vi "Teleop.vi"(10 "Match Info":T4={"Autonomous Elapsed Seconds"=0.0, "TeleOp Elapsed Seconds"=0.0, "Disabled Elapsed Seconds"=0.0, "Visited Autonomous"=FALSE, "Visited TeleOp"=FALSE, "Visited Disabled"=FALSE, "Autonomous Settings"={"Autonomous Style"=enum."Independent", "VI Refnum"=refnum}}, 11 "Call Context":T5) -> ()   [LabVIEW 2016]
doc: "This VI is called for each TeleOp packet received from the DS where the robot is not disabled. It is often used to read from the joysticks and update I/O or to update setpoints for timed control loops. It should complete and return within 20 milliseconds or it may miss DS packets."
uses:
  <vilib>/Rock Robotics/WPI/DriverStation/WPI_DriverStationDerivedRobotMode.ctl
  <vilib>/Rock Robotics/WPI/DriverStation/WPI_DriverStationMatch Info.ctl
  <vilib>/Rock Robotics/WPI/ThirdParty/CanMotor/TalonSRX/CTRE_CANTalonSRX_VelocityMeasurementPeriod.ctl
  <vilib>/Rock Robotics/WPI/ThirdParty/CanMotor/TalonSRX/WPI_CANTalonSRX_BrakeOverride.ctl
  <vilib>/Rock Robotics/WPI/ThirdParty/CanMotor/TalonSRX/WPI_CANTalonSRX_APIControlMode.ctl
  <vilib>/Rock Robotics/WPI/Utilities/WPI_GetSetVariantRefNum.vi
  <vilib>/Rock Robotics/Network Tables/NT Write Numeric Array.vi
  <vilib>/Rock Robotics/Network Tables/NT Write Boolean Array.vi
  <vilib>/Rock Robotics/Network Tables/NT Write Number.vi
  <vilib>/Rock Robotics/Network Tables/NT Read Boolean.vi
  <vilib>/Rock Robotics/Network Tables/NT Read Number.vi
  Robot Global Data.vi
panel:
  in  "Gear speed":dbl=2.0
  in  "Servo Disengaged Pos":dbl
  in  "Servo Engaged Pos":dbl
  in  "Disable Flash":bool=TRUE
  out "Display Mode":T1(ring)
  out "Color":T2(ring)
  out "Servo Position":dbl
  out "Error Left":dbl
  out "Error Right":dbl
  in  "P Shooting":dbl=0.08
  in  "Shooter \n%VBus":dbl
  out "Left Drive RPM":cluster{"Sensor Velocity":dbl, dbl}(graph)
  out "Right Drive RPM":cluster{"Sensor Velocity":dbl, dbl}(graph)
  out "Left RPM":dbl
  out "Right RPM":dbl
  in  "Shoot":bool
  out "DISABLED":bool
  out "Right FPS":dbl
  out "Left FPS":dbl
  in  "Velocity Measurement Period":T3=1 items=["Period_1ms"=1, "Period_2ms"=2, "Period_5ms"=5, "Period_10ms"=10, "Period_20ms"=20, "Period_25ms"=25, "Period_50ms"=50, "Period_100ms"=100]
  in  "Velocity Sample Window":u32=100
  out "Background":bool
  out "Shooter RPM":dbl
  out "Velocity":cluster{"Sensor Velocity":dbl, "Output":dbl}(graph)
  in  "P":dbl=0.0125
  in  "I":dbl
  in  "D":dbl
  in  "F":dbl=0.167
  in  "I Zone":dbl
  in  "Ramp Rate":dbl
  # "Shooter Speed Settings"
  # "Shooter Options"
  # "LED Status"
  # "Servo"
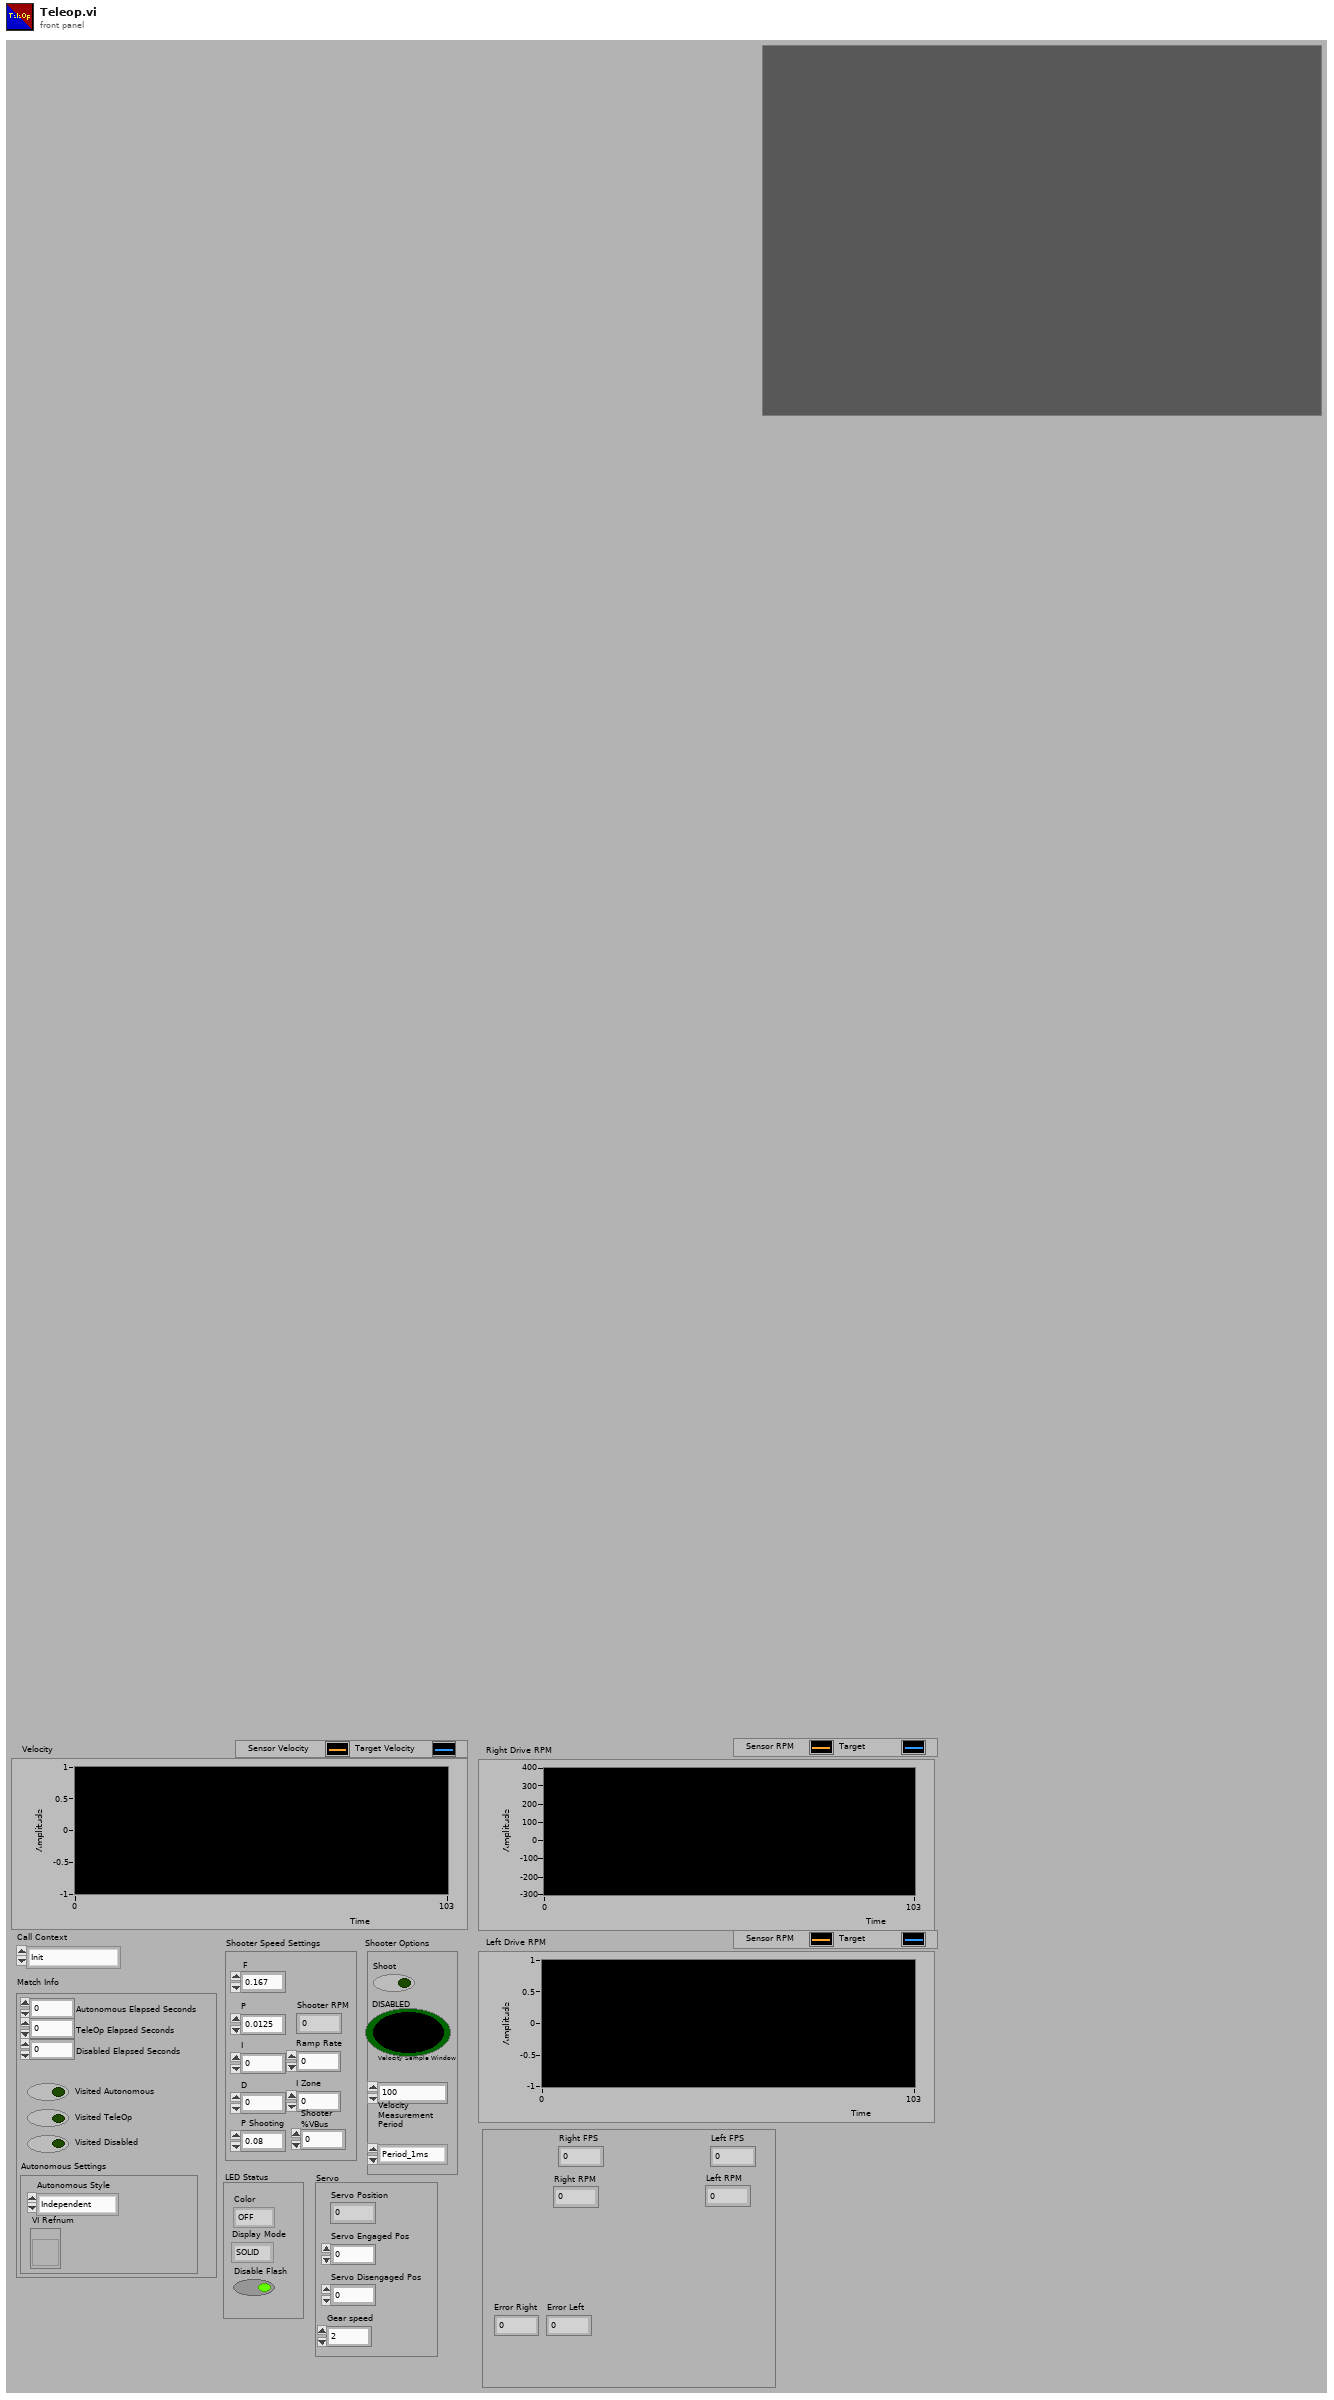
[diagram p1: front panel]
types:
  T1 = enum16{"SOLID", "FLASH 500ms", "FLASH 1000ms", "OFF"}
  T2 = enum16{"OFF", "RED", "GREEN", "BLUE", "PURPLE", "YELLOW", "TEAL", "WHITE", "RAINBOW"}
  T3 = typedef "CTRE_CANTalonSRX_VelocityMeasurementPeriod.ctl" = u16
  T4 = typedef "WPI_DriverStationMatch Info.ctl" = cluster{"Autonomous Elapsed Seconds":dbl, "TeleOp Elapsed Seconds":dbl, "Disabled Elapsed Seconds":dbl, "Visited Autonomous":bool, "Visited TeleOp":bool, "Visited Disabled":bool, "Autonomous Settings":cluster{"Autonomous Style":enum16{"Iterative", "Independent"}, "VI Refnum":refnum<vi>}}
  T5 = typedef "WPI_DriverStationDerivedRobotMode.ctl" = enum16{"Init", "Execute", "Stop"}
  T6 = typedef "WPI_CANTalonSRX_APIControlMode.ctl" = enum8{"Percent VBus", "Speed", "Position", "Slave", "Unchanged / Invalid", "Voltage Compensation", "Current", "Motion Profile", "Motion Magic"}
  T7 = typedef "WPI_CANTalonSRX_BrakeOverride.ctl" = enum8{"No Override", "Override to Coast", "Override to Brake"}
  T8 = cluster{"Shooter":cluster{"Shoot":bool, "%VBus":dbl, "Shoot Trigger":dbl, "Target Rpm":dbl}, "Drive":cluster{"Drive Stright":bool, "Left Throttle":dbl, "Right Throttle":dbl, "Curve Power":dbl}, "Intake":cluster{"Invert":bool, "%VBus":dbl}, "Gear/Climb":cluster{"Invert":bool, "%VBus":dbl}, "Teleop Front Pannel":cluster{"Overide?":bool}}
  T9 = typedef "WPI_JoystickDevRef.ctl" = cluster{"Device":T10}
  T10 = typedef "WPI_JoystickDeviceEnum.ctl" = enum16{"USB 0", "USB 1", "USB 2", "USB 3", "USB 4", "USB 5"}
  T11 = typedef "CTRE_PigeonIMU_DeviceRef.ctl" = cluster{"DeviceStatus":errorcluster, "Device Number":u8, "Type":T12, "Device ID":u32}
  T12 = typedef "CTRE_PigeonIMU_ConnectionType.ctl" = u32
  T13 = typedef "CTRE_PigeonIMU_GlobalStatus.ctl" = cluster{"PigeonState":T14, "FusedHeading":cluster{"Heading":dbl, "Valid?":bool, "Fusing?":bool}, "YPR":cluster{"Yaw":dbl, "Pitch":dbl, "Roll":dbl}, "Compass":cluster{"Heading":dbl, "Magnitude":dbl, "Absolute Heading":dbl}, "Accelerometer":cluster{"Biased":cluster{"X":i16, "Y":i16, "Z":i16, "Norm":i16}, "Angles":cluster{"XZ Tilt":dbl, "YZ Tilt":dbl, "XY Tilt":dbl}}, "Magnetometer":cluster{"Raw":cluster{"X":i16, "Y":i16, "Z":i16}, "Biased":cluster{"X":i16, "Y":i16, "Z":i16}}, "Gyro":cluster{"X":dbl, "Y":dbl, "Z":dbl, "Norm":dbl}, "6D Quaternian":cluster{"W":dbl, "X":dbl, "Y":dbl, "Z":dbl}, "Temp. (C)":dbl, "UpTime":u32, "StartupStatus":cluster{"ResetCount":i32, "ResetFlags":i32, "FirmwareVersion":i32, "HasReset?":bool}, "Calibration":cluster{"CurrentMode":T15, "LastCalError":i32, "CalBooting?":bool}, "CAN Error":errorcluster, "AccumGyro":cluster{"X":dbl, "Y":dbl, "Z":dbl}, "Usage Frame":u32}
  T14 = typedef "CTRE_PigeonIMU_PigeonState.ctl" = enum16{"NoComm", "Initializing", "Ready", "UserCalibration"}
  T15 = typedef "CTRE_PigeonIMU_CalibrationMode.ctl" = u16
  T16 = typedef "WPI_PotentiometerDevRef.ctl" = cluster{"DevStatus":errorcluster, "Analog Channel":T17, "Invert Output":bool}
  T17 = typedef "FPGA_AIChannel.ctl" = enum8{"AI 0", "AI 1", "AI 2", "AI 3", "AI MXP 0", "AI MXP 1", "AI MXP 2", "AI MXP 3", "Invalid"}
  T18 = typedef "WPI_MotorControlDeviceRef.ctl" = cluster{"DeviceStatus":errorcluster, "Type":T19, "PWM":cluster{"PWM Channel":T20, "DeadBand":T21}, "CAN":cluster{"Device Number":u8, "SetOutput VI Ref":variant, "GetOutput VI Ref":variant, "Enable VI Ref":variant, "Disable VI Ref":variant, "Data":variant}, "Invert":bool}
  T19 = typedef "WPI_MotorControlType.ctl" = enum16{"PWM", "CAN"}
  T20 = typedef "FPGA_DIOPWMChannel.ctl" = enum8{"PWM 0", "PWM 1", "PWM 2", "PWM 3", "PWM 4", "PWM 5", "PWM 6", "PWM 7", "PWM 8", "PWM 9", "PWM MXP 0", "PWM MXP 1", "PWM MXP 2", "PWM MXP 3", "PWM MXP 4", "PWM MXP 5", "PWM MXP 6", "PWM MXP 7", "PWM MXP 8", "PWM MXP 9", "Invalid"}
  T21 = typedef "WPI_PWMDeadband.ctl" = cluster{"Name":string, "maxPositivePwm":i32, "minPositivePwm":i32, "centerPwm":i32, "maxNegativePwm":i32, "minNegativePwm":i32, "angularRange":u16}
  T22 = typedef "WPI_ServoDeviceRef.ctl" = cluster{"DeviceStatus":errorcluster, "PWM Channel":T20, "DeadBand":T21}
  T23 = typedef "WPI_CANTalonSRX_GlobalStatus.ctl" = cluster{"Applied Throttle":dbl, "Module Enabled":bool, "CAN Error":errorcluster, "Closed Loop Error":dbl, "Forward Limit Switch Closed":bool, "Reverse Limit Switch Closed":bool, "Sensor Position":dbl, "Sensor Velocity":dbl, "Current":dbl, "Sticky Fault - Over Temp":bool, "Sticky Fault - Under Voltage":bool, "Sticky Fault - Forward Limit":bool, "Sticky Fault - Reverse Limit":bool, "Sticky Fault - Forward Soft Limit":bool, "Sticky Fault - Reverse Soft Limit":bool, "Brake is Enabled":bool, "Encoder Position":dbl, "Encoder Velocity":dbl, "Encoder Index Count":dbl, "Encoder A Pin State":bool, "Encoder B Pin State":bool, "Encoder Index Pin State":bool, "Analog In":dbl, "Analog In Velocity":dbl, "Temperature (C)":dbl, "Battery Voltage":dbl, "Control 5 Is Supported":bool, "Current Profile Slot Select":dbl, "Pos Div 8":bool, "Vel Div 4":bool, "Pulse Width Position":i32, "Pulse Width Velocity":i32, "Pulse Width Rise To Rise (us)":i32, "Pulse Width Rise To Fall (us)":i32, "Mot Prof Active Is Under Run":bool, "Mot Prof Active Has Under Run":bool, "Mot Prof Active Is Last":bool, "Mot Prof Active Velocity Only":bool, "Mot Prof Active Is Valid":bool, "Mot Prof Buffer Is Full":bool, "Mot Prof Active Profile Slot Select":i32, "Mot Prof NextID":i32, "Mot Prof Count":i32, "Mot Prof Active Velocity":dbl, "Mot Prof Active Position":dbl, "Mot Prof Output Enable":i32, "UsageFrame":u32, "Motion Magic Active Trajectory":cluster{"Velocity":dbl, "Position":dbl}}
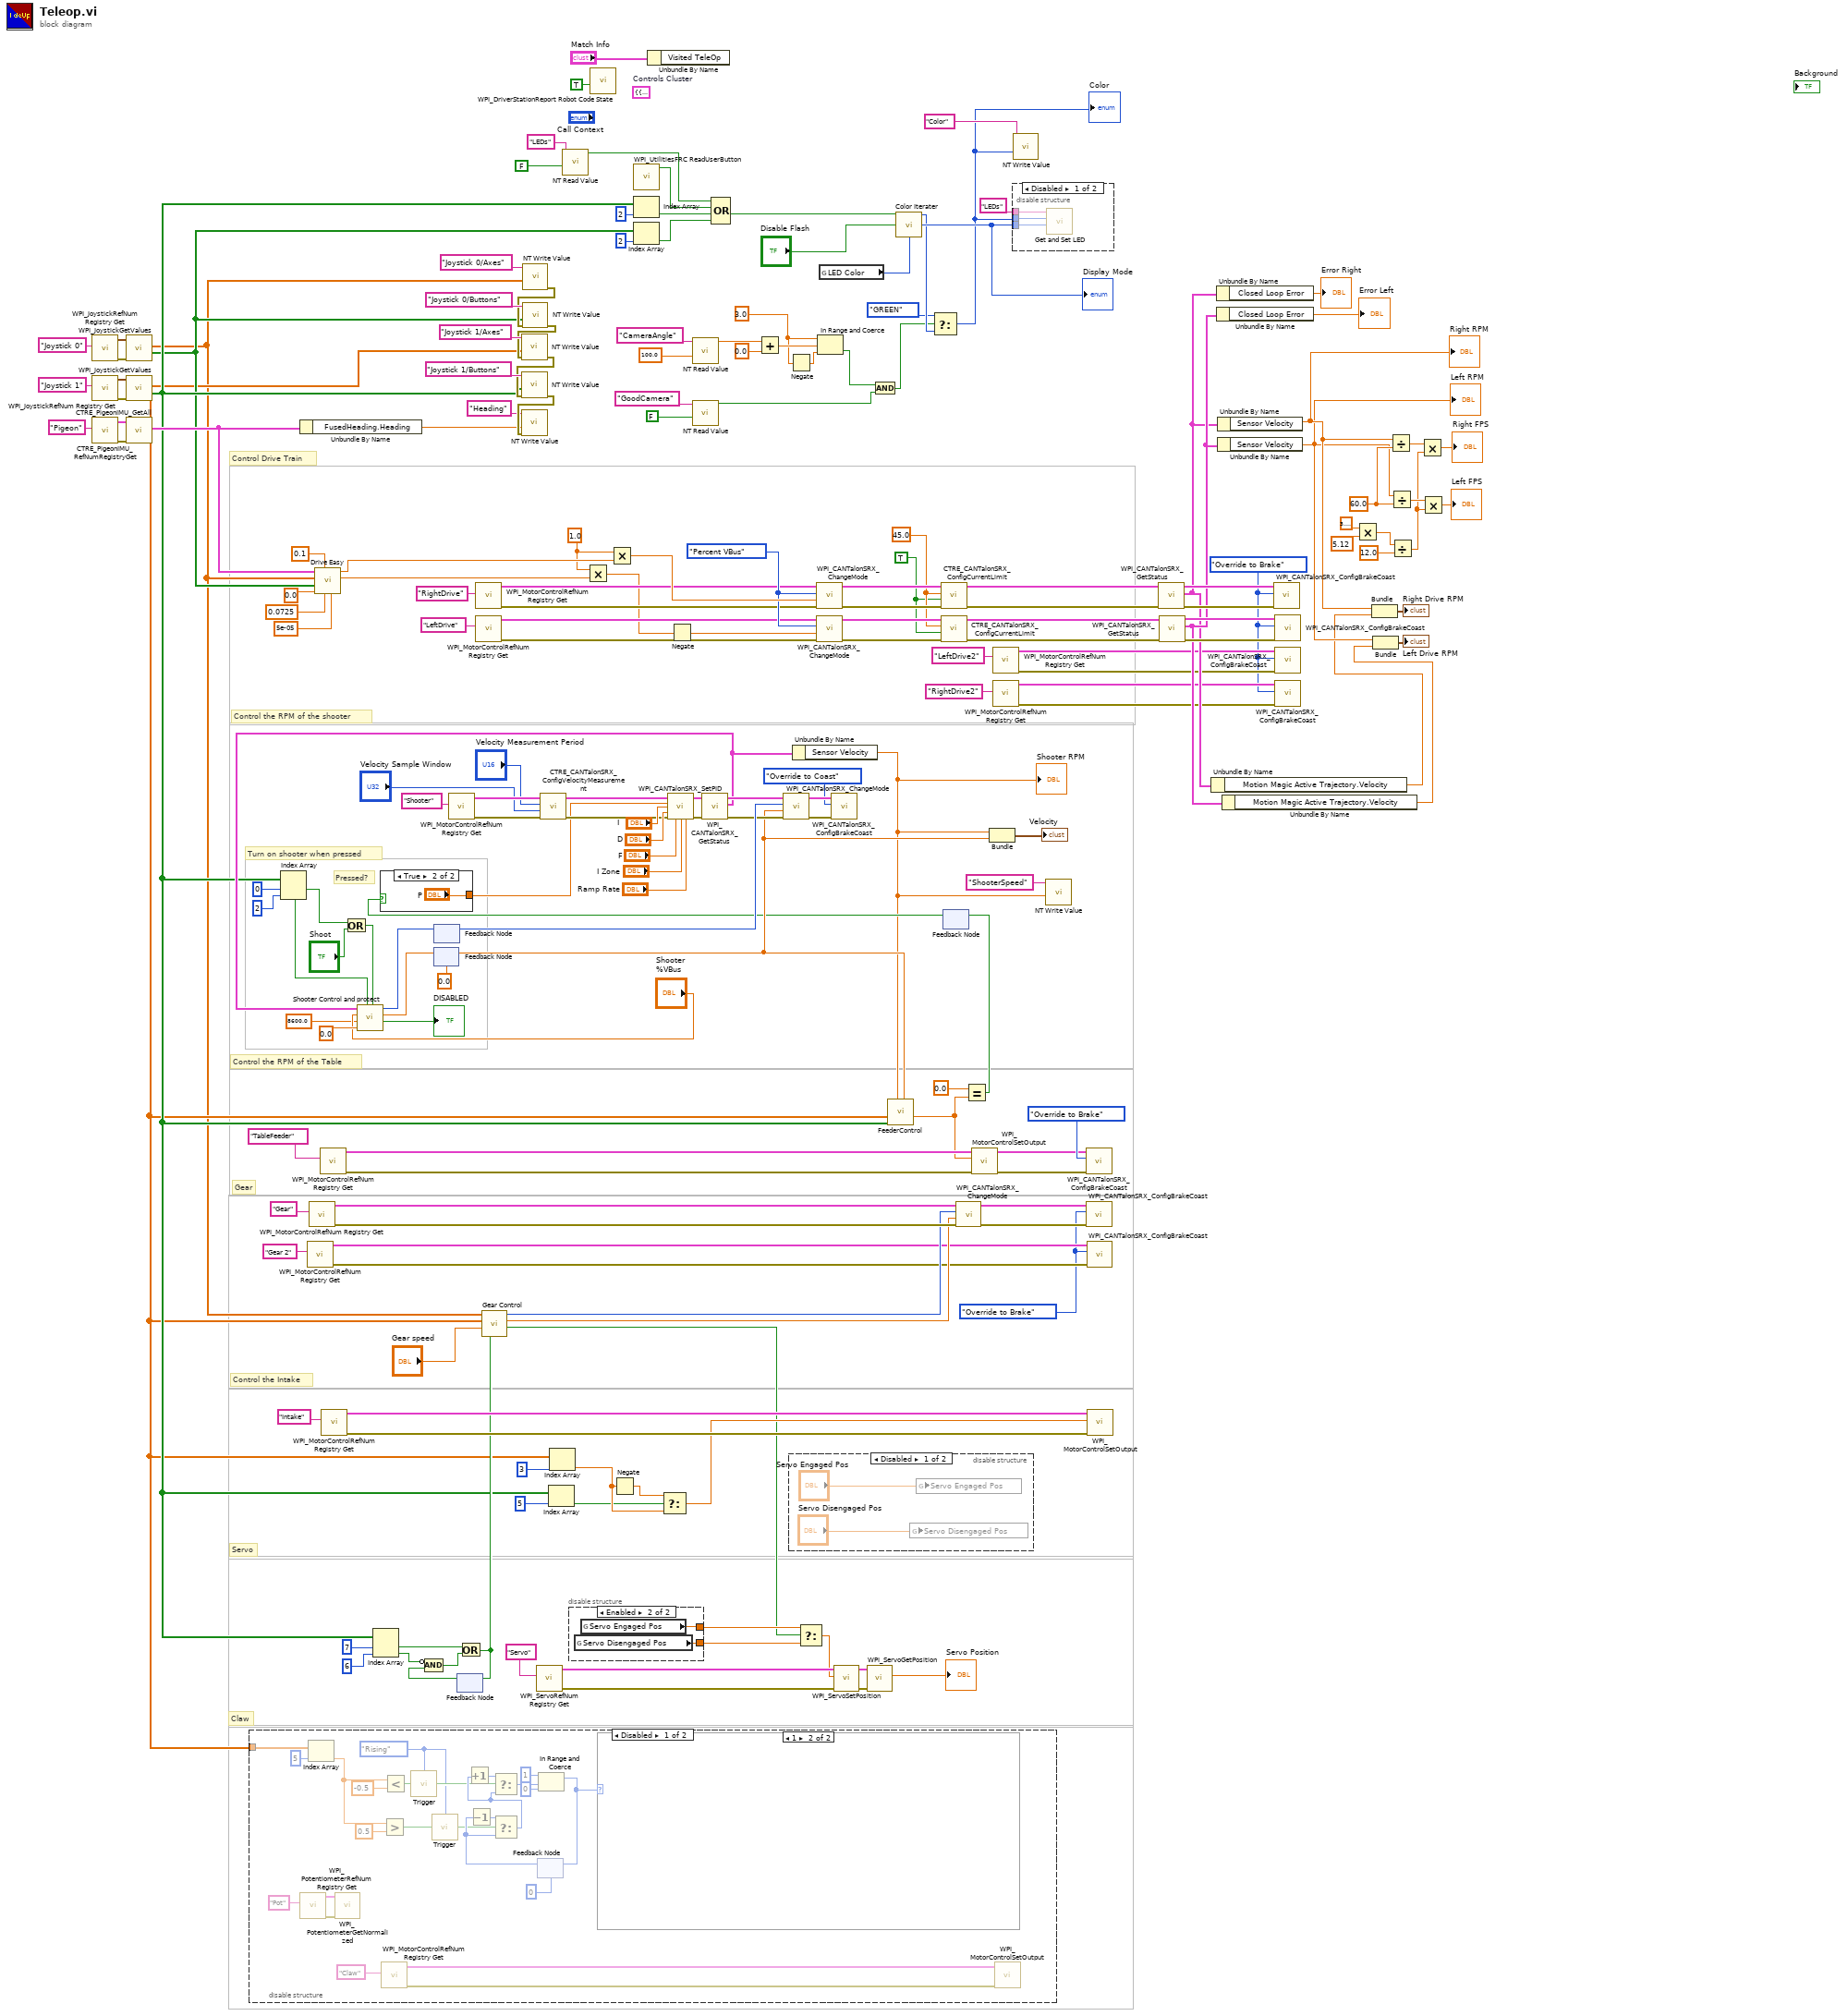
[diagram p0: block diagram]
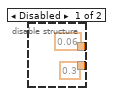
[diagram p4: hidden frame]
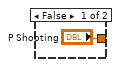
[diagram p7: hidden frame]
diagram:
  w1 = 1.0 ("x")
  w139 = WPI_CANTalonSRX_APIControlMode."Percent VBus" ("Control Mode")
  w5 = 3.0 ("upper limit")
  w28 = WPI_CANTalonSRX_BrakeOverride."Override to Brake" ("Brake / Coast Mode")
  w32 = WPI_CANTalonSRX_BrakeOverride."Override to Brake" ("Brake / Coast Mode")
  w73 = TRUE ("Enable Current Limit?")
  w74 = 45.0 ("Current Limit (Amps)")
  w134 = 60.0 ("y")
  (unwired) T8 {"Shooter"={"Shoot"=FALSE, "%VBus"=0.0, "Shoot Trigger"=0.0, "Target Rpm"=0.0}, "Drive"={"Drive Stright"=FALSE, "Left Throttle"=0.0, "Right Throttle"=0.0, "Curve Power"=0.0}, "Intake"={"Invert"=FALSE, "%VBus"=0.0}, "Gear/Climb"={"Invert"=FALSE, "%VBus"=0.0}, "Teleop Front Pannel"={"Overide?"=FALSE}}  # Controls Cluster
  # "Claw"
  # "Servo"
  # "Pressed?"
  # "Gear"
  # "Turn on shooter when pressed"
  # "Control the Intake"
  # "Control the RPM of the Table"
  # "Control the RPM of the shooter"
  # "Control Drive Train"
  n1 = call <vilib>:"WPI_JoystickRefNum Registry Get.vi"("refnum name"="Joystick 0") -> ("error out"=w195:errorcluster, "JoystickDevRef"=w183:T9)  [unwired: 1 in, 8 out]
  n2 = call <vilib>:"WPI_JoystickRefNum Registry Get.vi"("refnum name"="Joystick 1") -> ("error out"=w185:errorcluster, "JoystickDevRef"=w190:T9)  [unwired: 1 in, 8 out]
  n3 = call <vilib>:"CTRE_PigeonIMU_RefNumRegistryGet.vi"("refnum name"="Pigeon") -> ("error out"=w180:errorcluster, "PigeonIMUDevRef"=w181:T11)  [unwired: 9 in]
  n4 = call <vilib>:"WPI_JoystickGetValues.vi"("error in (no error)"=w195, "JoystickDevRef"=w183) -> ("Buttons"=w43:bool[], "Axes"=w20:dbl[])  [unwired: 5 in, 3 out]
  n5 = call <vilib>:"WPI_JoystickGetValues.vi"("error in (no error)"=w185, "JoystickDevRef"=w190) -> ("Buttons"=w56:bool[], "Axes"=w21:dbl[])  [unwired: 5 in, 3 out]
  n6 = call <vilib>:"CTRE_PigeonIMU_GetAll.vi"("error in (no error)"=w180, "PigeonIMUDevRef"=w181) -> ("Get All"=w176:T13)  [unwired: 7 in, 2 out]
  n7 = disable-structure shown="Disabled" {
    disable-tunnel: w21 -> [w219 _]
    frame Disabled {
      w202 = enum16{"Falling", "Rising", "Both"}."Rising" ("Enum")
      n8 = call <vilib>:"WPI_PotentiometerRefNum Registry Get.vi"("refnum name"="Pot") -> ("error out"=w221:errorcluster, "PotDevRef"=w220:T16)  [unwired: 9 in]
      n9 = Index Array(array=w219, index=5) -> (element=w216:dbl)
      n10 = call <vilib>:"WPI_PotentiometerGetNormalized.vi"("error in"=w221, "PotDevRef"=w220) -> ()  [unwired: 7 in, 3 out]
      n11 = call <vilib>:"WPI_MotorControlRefNum Registry Get.vi"("refnum name"="Claw") -> ("error out"=w224:errorcluster, "MotorControlDevRef"=w223:T18)  [unwired: 9 in]
      n12 = Greater?(x=w216, y=0.5) -> (0:w206:bool)
      n13 = Less?(x=w216, y=-0.5) -> (x < y?=w204:bool)
      n14 = call "Trigger.vi"("Enum"=w202, "Button"=w204) -> ("Trigger"=w203:bool)  [unwired: 13 in]
      n15 = call "Trigger.vi"("Enum"=w202, "Button"=w206) -> ("Trigger"=w205:bool)  [unwired: 13 in]
      n16 = feedback #1(0) -> (w209:i32)
      n17 = Decrement(x=w209) -> (x-1=w210:i32)
      n18 = Select(t=w210, s=w205, f=w209) -> (s? t:f=w207:i32)
      n19 = Increment(x=w207) -> (x+1=w208:i32)
      n20 = Select(t=w208, s=w203, f=w207) -> (s? t:f=w214:i32)
      n21 = In Range and Coerce(upper limit=1, x=w214, lower limit=0) -> (coerced(x)=w201:i32)  [unwired: 1 out]
      n22 = feedback-in #1(w201) -> ()
      n23 = case shown="1" w201 {
        frame 0, Default {
        }
        frame 1 {
        }
      }
      n24 = call <vilib>:"WPI_MotorControlSetOutput.vi"("error in (no error)"=w224, "MotorControlDevRef"=w223) -> ()  [unwired: 7 in, 3 out]
    }
    frame Enabled {
    }
  }
  n25 = Index Array(array=w56, index #1=0 ("index"), index #2=2 ("index")) -> (element #1=w94:bool, element #2=w92:bool)
  n26 = Unbundle By Name(w176) -> ("FusedHeading.Heading"=w177:dbl)
  n27 = call <vilib>:"WPI_MotorControlRefNum Registry Get.vi"("refnum name"="Gear 2") -> ("error out"=w40:errorcluster, "MotorControlDevRef"=w39:T18)  [unwired: 9 in]
  n28 = call <vilib>:"WPI_MotorControlRefNum Registry Get.vi"("refnum name"="Gear") -> ("error out"=w107:errorcluster, "MotorControlDevRef"=w108:T18)  [unwired: 9 in]
  n29 = call "Drive Easy.vi"("D Gain"=5e-05, "P Gain"=0.0725, "Automatic Drive Stright Range"=0.1, "Operator"=0.0 ("Curve"), "Buttons"=w43, "Axes"=w20, "Get All"=w176) -> ("Left Motor Value"=w140:dbl, "Right Motor Value"=w141:dbl)  [unwired: 2 in, 1 out]
  n30 = call <vilib>:"WPI_MotorControlRefNum Registry Get.vi"("refnum name"="TableFeeder") -> ("error out"=w168:errorcluster, "MotorControlDevRef"=w169:T18)  [unwired: 9 in]
  n31 = call <vilib>:"WPI_MotorControlRefNum Registry Get.vi"("refnum name"="Intake") -> ("error out"=w116:errorcluster, "MotorControlDevRef"=w117:T18)  [unwired: 9 in]
  n32 = Or(x=w94, y="Shoot") -> (x .or. y?=w150:bool)
  n33 = Index Array(array=w56, index #1=7 ("index"), index #2=6 ("index")) -> (element #1=w71:bool, element #2=w59:bool)
  n34 = feedback #2(0.0 ("Output")) -> (w125:dbl)
  n35 = feedback #3() -> (w151:T6)  [unwired: 1 in]
  n36 = call <vilib>:"WPI_MotorControlRefNum Registry Get.vi"("refnum name"="Shooter") -> ("error out"=w174:errorcluster, "MotorControlDevRef"=w175:T18)  [unwired: 9 in]
  n37 = feedback #4() -> (w58:bool)  [unwired: 1 in]
  n38 = Compound Arithmetic op=AND(invert w59, w58) -> (w57:bool)
  n39 = Or(x=w71, y=w57) -> (x .or. y?=w65:bool)
  n40 = feedback-in #4(w65) -> ()
  n41 = call <vilib>:"WPI_MotorControlRefNum Registry Get.vi"("refnum name"="RightDrive") -> ("error out"=w119:errorcluster, "MotorControlDevRef"=w118:T18)  [unwired: 9 in]
  n42 = call <vilib>:"WPI_MotorControlRefNum Registry Get.vi"("refnum name"="LeftDrive") -> ("error out"=w137:errorcluster, "MotorControlDevRef"=w138:T18)  [unwired: 9 in]
  n43 = call "Gear Control.vi"("Boolean"=w65, "Gear speed"="Gear speed", "Axes 2"=w21, "Axes"=w20) -> ("Output"=w60:bool, "upper limit"=w67:dbl, "Control Mode"=w66:T6)  [unwired: 5 in]
  n44 = call-poly <vilib>:"NT Write Value.vi"("Numeric Array"=w20, "Name"="Joystick 0/Axes") -> ("error out"=w194:errorcluster)  [unwired: 9 in]
  n45 = call-poly <vilib>:"NT Write Value.vi"("error in"=w194, "Boolean Array"=w43, "Name"="Joystick 0/Buttons") -> ("error out"=w184:errorcluster)  [unwired: 8 in]
  n46 = call-poly <vilib>:"NT Write Value.vi"("error in"=w184, "Numeric Array"=w21, "Name"="Joystick 1/Axes") -> ("error out"=w186:errorcluster)  [unwired: 8 in]
  n47 = call-poly <vilib>:"NT Write Value.vi"("error in"=w186, "Boolean Array"=w56, "Name"="Joystick 1/Buttons") -> ("error out"=w179:errorcluster)  [unwired: 8 in]
  n48 = call-poly <vilib>:"NT Write Value.vi"("error in"=w179, "Numeric"=w177, "Name"="Heading") -> ()  [unwired: 8 in, 1 out]
  n49 = call <vilib>:"WPI_ServoRefNum Registry Get.vi"("refnum name"="Servo") -> ("error out"=w64:errorcluster, "ServoDeviceRef"=w68:T22)  [unwired: 9 in]
  n50 = call <vilib>:"CTRE_CANTalonSRX_ConfigVelocityMeasurement.vi"("error in (no error)"=w174, "Velocity Sample Window"="Velocity Sample Window", "Velocity Measurement Period"="Velocity Measurement Period", "CAN Talon SRX Ref"=w175) -> ("error out"=w159:errorcluster, "CAN Talon SRX Ref"=w158:T18)  [unwired: 6 in]
  n51 = Index Array(array=w56, index=5) -> (element=w102:bool)
  n52 = Index Array(array=w21, index=3) -> (element=w103:dbl)
  n53 = call-poly <vilib>:"NT Read Value.vi"("Default Value"=FALSE, "Name"="LEDs") -> ("Boolean"=w25:bool)  [unwired: 8 in, 1 out]
  n54 = disable-structure shown="Enabled" {
    disable-tunnel: [0.06 ("t") w229] -> w63
    disable-tunnel: [0.3 ("f") w228] -> w62
    frame Disabled {
    }
    frame Enabled {
      n55 = global read "Robot Global Data.vi" "Servo Disengaged Pos"() -> (w228:dbl)
      n56 = global read "Robot Global Data.vi" "Servo Engaged Pos"() -> (w229:dbl)
    }
  }
  n57 = Multiply(x=w1, y=w140) -> (x*y=w2:dbl)
  n58 = call <vilib>:"WPI_DriverStationReport Robot Code State.vi"("TeleOp"=TRUE ("Autonomous")) -> ()  [unwired: 10 in, 1 out]
  n59 = Multiply(x=w1, y=w141) -> (x*y=w143:dbl)
  n60 = Negate(x=w103) -> (-x=w104:dbl)
  n61 = call <vilib>:"WPI_UtilitiesFRC ReadUserButton.vi"() -> ("User Button"=w48:bool)  [unwired: 10 in, 1 out]
  n62 = Index Array(array=w56, index=2) -> (element=w47:bool)
  n63 = Index Array(array=w43, index=2) -> (element=w44:bool)
  n64 = Unbundle By Name("Match Info") -> ()  [unwired: 1 out]
  n65 = Select(t=w104, s=w102, f=w103) -> (s? t:f=w105:dbl)
  n66 = Negate(x=w2) -> (-x=w142:dbl)
  n67 = call-poly <vilib>:"NT Read Value.vi"("Default Value"=100.0, "Name"="CameraAngle") -> ("Numeric"=w8:dbl)  [unwired: 8 in, 1 out]
  n68 = call-poly <vilib>:"NT Read Value.vi"("Default Value"=FALSE, "Name"="GoodCamera") -> ("Boolean"=w10:bool)  [unwired: 8 in, 1 out]
  n69 = Compound Arithmetic op=OR(w25, w48, w47, w44) -> (w46:bool)
  n70 = Add(x=w8, y=0.0) -> (x+y=w9:dbl)
  n71 = Negate(x=w5) -> (-x=w6:dbl)
  n72 = disable-structure shown="Disabled" {
    frame Disabled {
      n73 = global write "Robot Global Data.vi" "Servo Disengaged Pos"("Servo Disengaged Pos") -> ()
      n74 = global write "Robot Global Data.vi" "Servo Engaged Pos"("Servo Engaged Pos") -> ()
    }
    frame Enabled {
    }
  }
  n75 = Select(t=w63, s=w60, f=w62) -> (s? t:f=w61:dbl)
  n76 = call <vilib>:"WPI_CANTalonSRX_ChangeMode.vi"("error in (no error)"=w119, "Output"=w143, "Control Mode"=w139, "CAN Talon SRX Ref"=w118) -> ("error out"=w82:errorcluster, "CAN Talon SRX Ref"=w81:T18)  [unwired: 6 in]
  n77 = call <vilib>:"WPI_CANTalonSRX_ChangeMode.vi"("error in (no error)"=w137, "Output"=w142, "Control Mode"=w139, "CAN Talon SRX Ref"=w138) -> ("error out"=w77:errorcluster, "CAN Talon SRX Ref"=w78:T18)  [unwired: 6 in]
  n78 = In Range and Coerce(upper limit=w5, x=w9, lower limit=w6) -> (In Range?=w4:bool)  [unwired: 1 out]
  n79 = global read "Robot Global Data.vi" "LED Color"() -> (w27:T2)
  n80 = call <vilib>:"WPI_ServoSetPosition.vi"("error in (no error)"=w64, "Position"=w61, "ServoDeviceRef"=w68) -> ("error out"=w69:errorcluster, "ServoDeviceRef"=w70:T22)  [unwired: 7 in]
  n81 = call <vilib>:"WPI_ServoGetPosition.vi"("error in (no error)"=w69, "ServoDeviceRef"=w70) -> ("Position"=→"Servo Position":dbl)  [unwired: 7 in, 2 out]
  n82 = And(x=w4, y=w10) -> (x .and. y?=w11:bool)
  n83 = call "Color Iterater.vi"("Change Color"=w46, "Disable Flash"="Disable Flash", "Initial Color"=w27) -> ("Color"=w17:T2, "Display Mode"=w41:T1)  [unwired: 11 in]
  "Display Mode" <- w41
  n84 = Select(t=T2."GREEN", s=w11, f=w17) -> (s? t:f=w18:T2)
  "Color" <- w18
  n85 = call <vilib>:"CTRE_CANTalonSRX_ConfigCurrentLimit.vi"("error in (no error)"=w82, "Enable Current Limit?"=w73, "Current Limit (Amps)"=w74, "CAN Talon SRX Ref"=w81) -> ("error out"=w79:errorcluster, "CAN Talon SRX Ref"=w80:T18)  [unwired: 6 in]
  n86 = call <vilib>:"CTRE_CANTalonSRX_ConfigCurrentLimit.vi"("error in (no error)"=w77, "Enable Current Limit?"=w73, "Current Limit (Amps)"=w74, "CAN Talon SRX Ref"=w78) -> ("error out"=w76:errorcluster, "CAN Talon SRX Ref"=w75:T18)  [unwired: 6 in]
  n87 = feedback #5() -> (w112:bool)  [unwired: 1 in]
  n88 = case shown="True" w112 {
    tunnel: ["P Shooting" "P"] -> w115
    frame False {
    }
    frame True {
    }
  }
  n89 = call <vilib>:"WPI_CANTalonSRX_SetPID.vi"("CAN Talon SRX Ref"=w158, "P"=w115, "I"="I", "D"="D", "error in (no error)"=w159, "F"="F", "I Zone"="I Zone", "Ramp Rate"="Ramp Rate") -> ("CAN Talon SRX Ref"=w148:T18, "error out"=w147:errorcluster)  [unwired: 6 in]
  n90 = call <vilib>:"WPI_CANTalonSRX_GetStatus.vi"("error in (no error)"=w147, "CAN Talon SRX Ref"=w148) -> ("error out"=w146:errorcluster, "Talon SRX Status"=w126:T23, "CAN Talon SRX Ref"=w145:T18)  [unwired: 7 in]
  n91 = call "Shooter Control and protect.vi"("Shoot"=w150, "Reset"=w92, "Auto Reset Delay (ms)"=0.0 ("Auto Reset Delay"), "Target RPM"=8600.0, "%VBus"="Shooter \n%VBus", "Talon Status"=w126) -> ("DISABLED"=→"DISABLED":bool, "Output"=w153:dbl, "Control Mode"=w152:T6)  [unwired: 3 in]
  n92 = feedback-in #2(w153) -> ()
  n93 = feedback-in #3(w152) -> ()
  n94 = call <vilib>:"WPI_CANTalonSRX_ChangeMode.vi"("error in (no error)"=w146, "Output"=w125, "Control Mode"=w151, "CAN Talon SRX Ref"=w145) -> ("error out"=w31:errorcluster, "CAN Talon SRX Ref"=w30:T18)  [unwired: 6 in]
  n95 = Unbundle By Name(w126) -> ("Sensor Velocity"=w89:dbl)
  "Shooter RPM" <- w89
  n96 = call <vilib>:"WPI_CANTalonSRX_ConfigBrakeCoast.vi"("error in (no error)"=w31, "Brake / Coast Mode"=WPI_CANTalonSRX_BrakeOverride."Override to Coast", "CAN Talon SRX Ref"=w30) -> ()  [unwired: 7 in, 2 out]
  n97 = call "FeederControl.vi"("Target RPM"=w125, "RPM"=w89, "Buttons"=w56, "Axes"=w21) -> ("Output"=w114:dbl)  [unwired: 6 in, 1 out]
  n98 = call <vilib>:"WPI_CANTalonSRX_ChangeMode.vi"("error in (no error)"=w107, "Output"=w67, "Control Mode"=w66, "CAN Talon SRX Ref"=w108) -> ("error out"=w36:errorcluster, "CAN Talon SRX Ref"=w37:T18)  [unwired: 6 in]
  n99 = Equal?(x=0.0, y=w114) -> (x = y?=w113:bool)
  n100 = feedback-in #5(w113) -> ()
  n101 = call <vilib>:"WPI_MotorControlSetOutput.vi"("error in (no error)"=w168, "Output"=w114, "MotorControlDevRef"=w169) -> ("error out"=w33:errorcluster, "MotorControlDevRef"=w34:T18)  [unwired: 6 in, 1 out]
  n102 = Bundle("Sensor Velocity"=w89, "Output"=w125) -> (→"Velocity":cluster{"Sensor Velocity":dbl, "Output":dbl})  [unwired: 1 in]
  n103 = call <vilib>:"WPI_MotorControlRefNum Registry Get.vi"("refnum name"="LeftDrive2") -> ("error out"=w50:errorcluster, "MotorControlDevRef"=w51:T18)  [unwired: 9 in]
  n104 = call <vilib>:"WPI_MotorControlRefNum Registry Get.vi"("refnum name"="RightDrive2") -> ("error out"=w52:errorcluster, "MotorControlDevRef"=w53:T18)  [unwired: 9 in]
  n105 = disable-structure shown="Disabled" {
    disable-tunnel: "LEDs" -> [w236 _]
    disable-tunnel: w41 -> [w235 _]
    disable-tunnel: w18 -> [w234 _]
    frame Disabled {
      n106 = call "Get and Set LED.vi"("Display Mode"=w235, "Color"=w234, "refnum name"=w236) -> ()  [unwired: 9 in]
    }
    frame Enabled {
    }
  }
  n107 = call-poly <vilib>:"NT Write Value.vi"("Numeric"=w18, "Name"="Color") -> ()  [unwired: 9 in, 1 out]
  n108 = call-poly <vilib>:"NT Write Value.vi"("Numeric"=w89, "Name"="ShooterSpeed") -> ()  [unwired: 9 in, 1 out]
  n109 = call <vilib>:"WPI_CANTalonSRX_ConfigBrakeCoast.vi"("error in (no error)"=w33, "Brake / Coast Mode"=WPI_CANTalonSRX_BrakeOverride."Override to Brake", "CAN Talon SRX Ref"=w34) -> ()  [unwired: 7 in, 2 out]
  n110 = call <vilib>:"WPI_CANTalonSRX_ConfigBrakeCoast.vi"("error in (no error)"=w36, "Brake / Coast Mode"=w32, "CAN Talon SRX Ref"=w37) -> ()  [unwired: 7 in, 2 out]
  n111 = call <vilib>:"WPI_CANTalonSRX_ConfigBrakeCoast.vi"("error in (no error)"=w40, "Brake / Coast Mode"=w32, "CAN Talon SRX Ref"=w39) -> ()  [unwired: 7 in, 2 out]
  n112 = call <vilib>:"WPI_MotorControlSetOutput.vi"("error in (no error)"=w116, "Output"=w105, "MotorControlDevRef"=w117) -> ()  [unwired: 6 in, 3 out]
  n113 = call <vilib>:"WPI_CANTalonSRX_GetStatus.vi"("error in (no error)"=w79, "CAN Talon SRX Ref"=w80) -> ("error out"=w100:errorcluster, "Talon SRX Status"=w83:T23, "CAN Talon SRX Ref"=w101:T18)  [unwired: 7 in]
  n114 = call <vilib>:"WPI_CANTalonSRX_GetStatus.vi"("error in (no error)"=w76, "CAN Talon SRX Ref"=w75) -> ("error out"=w98:errorcluster, "Talon SRX Status"=w86:T23, "CAN Talon SRX Ref"=w99:T18)  [unwired: 7 in]
  n115 = Unbundle By Name(w83) -> ("Motion Magic Active Trajectory.Velocity"=w84:dbl)
  n116 = Unbundle By Name(w83) -> ("Closed Loop Error"=→"Error Right":dbl)
  n117 = Unbundle By Name(w86) -> ("Closed Loop Error"=→"Error Left":dbl)
  n118 = Unbundle By Name(w83) -> ("Sensor Velocity"=w123:dbl)
  "Right RPM" <- w123
  n119 = Unbundle By Name(w86) -> ("Sensor Velocity"=w122:dbl)
  "Left RPM" <- w122
  n120 = Unbundle By Name(w86) -> ("Motion Magic Active Trajectory.Velocity"=w85:dbl)
  n121 = call <vilib>:"WPI_CANTalonSRX_ConfigBrakeCoast.vi"("error in (no error)"=w100, "Brake / Coast Mode"=w28, "CAN Talon SRX Ref"=w101) -> ()  [unwired: 7 in, 2 out]
  n122 = call <vilib>:"WPI_CANTalonSRX_ConfigBrakeCoast.vi"("error in (no error)"=w98, "Brake / Coast Mode"=w28, "CAN Talon SRX Ref"=w99) -> ()  [unwired: 7 in, 2 out]
  n123 = call <vilib>:"WPI_CANTalonSRX_ConfigBrakeCoast.vi"("error in (no error)"=w50, "Brake / Coast Mode"=w28, "CAN Talon SRX Ref"=w51) -> ()  [unwired: 7 in, 2 out]
  n124 = call <vilib>:"WPI_CANTalonSRX_ConfigBrakeCoast.vi"("error in (no error)"=w52, "Brake / Coast Mode"=w28, "CAN Talon SRX Ref"=w53) -> ()  [unwired: 7 in, 2 out]
  n125 = Multiply(x=3.141592653589793, y=5.12) -> (x*y=w131:dbl)
  n126 = Bundle("Sensor Velocity"=w123, "Velocity"=w84) -> (→"Right Drive RPM":cluster{"Sensor Velocity":dbl, "Velocity":dbl})  [unwired: 1 in]
  n127 = Bundle("Sensor Velocity"=w122, "Velocity"=w85) -> (→"Left Drive RPM":cluster{"Sensor Velocity":dbl, "Velocity":dbl})  [unwired: 1 in]
  n128 = Divide(x=w123, y=w134) -> (x/y=w133:dbl)
  n129 = Divide(x=w122, y=w134) -> (x/y=w132:dbl)
  n130 = Divide(x=w131, y=12.0) -> (x/y=w130:dbl)
  n131 = Multiply(x=w133, y=w130) -> (x*y=→"Right FPS":dbl)
  n132 = Multiply(x=w132, y=w130) -> (x*y=→"Left FPS":dbl)
